vi "Digital Out Write.vi"(8 "error in (no error)":errorcluster, 10 "Port Mask":u64, 11 "SimSyA in":refnum<class "SimSyA.lvclass">) -> (0 "error out":errorcluster, 3 "SimSyA out":refnum<class "SimSyA.lvclass">)   [LabVIEW 2014, in "SimSyA.lvlib" / "SimSyA.lvclass"]
uses:
  SimSyA.lvclass
  SimSyA.lvclass/SimSyA.ctl
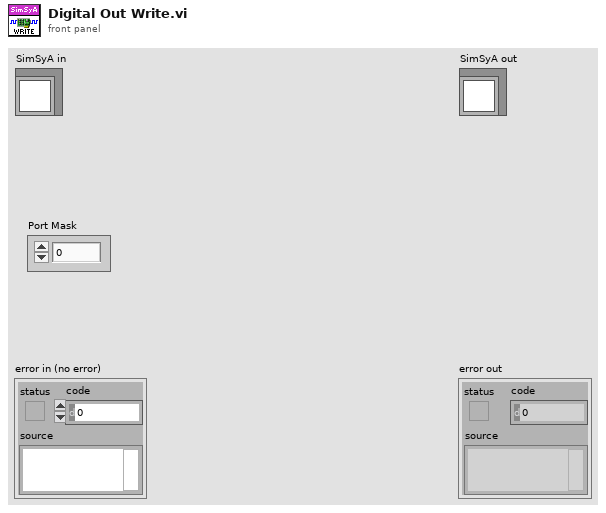
[diagram p1: front panel]
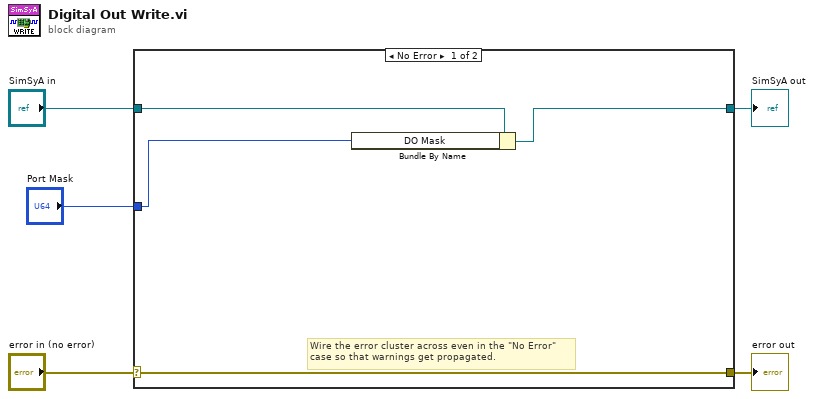
[diagram p0: block diagram]
diagram:
  n1 = case shown="No Error" "error in (no error)" {
    selector: "error in (no error)" -> [w9 w11]
    tunnel: [w9 w11] -> w4
    tunnel: [w7 w10] -> w2
    tunnel: "SimSyA in" -> [w8 w10]
    tunnel: "Port Mask" -> [w6 _]
    frame No Error {
      # "Wire the error cluster across even in the \"No Error\"\ncase so that warnings get propagated."
      n2 = Bundle By Name(cluster=w8, "DO Mask"=w6) -> (w7:refnum<class "SimSyA.lvclass">)
    }
    frame Error {
    }
  }
  "error out" <- w4
  "SimSyA out" <- w2
